vi "Status - Update Sequence Status.vi"(0 "Sequence Status":refnum<vi>, 1 "WPS Details":refnum<vi>, 2 "DB - Transaction":bool=TRUE, 3 "Transaction":T3, 5 "MCListBox FHS Setup":refnum<vi>, 7 "ET3504 Status":refnum<vi>, 11 "Error In":errorcluster, 12 "Parameter Cluster (Scaled)":T5={"ProgramNumber"=1, "CurProg"=33, "CurSeg"=1, "ProgStatus"=1, "ProgTimeLeft (min)"=0.0, "PVIn (degC)"=12000.0, "SPIn (NA)"=0.0, "SegTimeLeft (min)"=0.0}, 13 "DB - Active Process":bool=TRUE, 14 "Segment.Type":i16) -> (10 "Segment.Type II":i16, 15 "Error Out":errorcluster)   [LabVIEW 2013]
uses:
  Controls/Combo Box.ctl
  Controls/Transaction Cluster.ctl
  Controls/DB - Execute Transaction Enum.ctl
  Controls/DB - [TransactionResult] Enum.ctl
  Controls/DB - [Execute].[ActiveProcess] Enum.ctl
  Controls/DB - CMS Execute Active Process.ctl
  Controls/Global SRTRS.vi
panel:
  out "ET3504 Status":string="Offline."
  in  "WPS Details Setup 15":T2 caption="WPS Details"
  in  "MCListBox FHS Setup 2":i32(listbox) caption="Furnace Heating Sequence"
  out "Refnum error":errorcluster
  out "Seq-Seg Info":T4
  out "Sequence Status":string
  out "Total non-ZERO rows":i32
  # "Segment.Type\n0 - End\n1 - Rate\n3 - Dwell\n300 - mini Dwell"
  # "Segment.Type\n0 - End\n1 - Rate\n3 - Dwell"
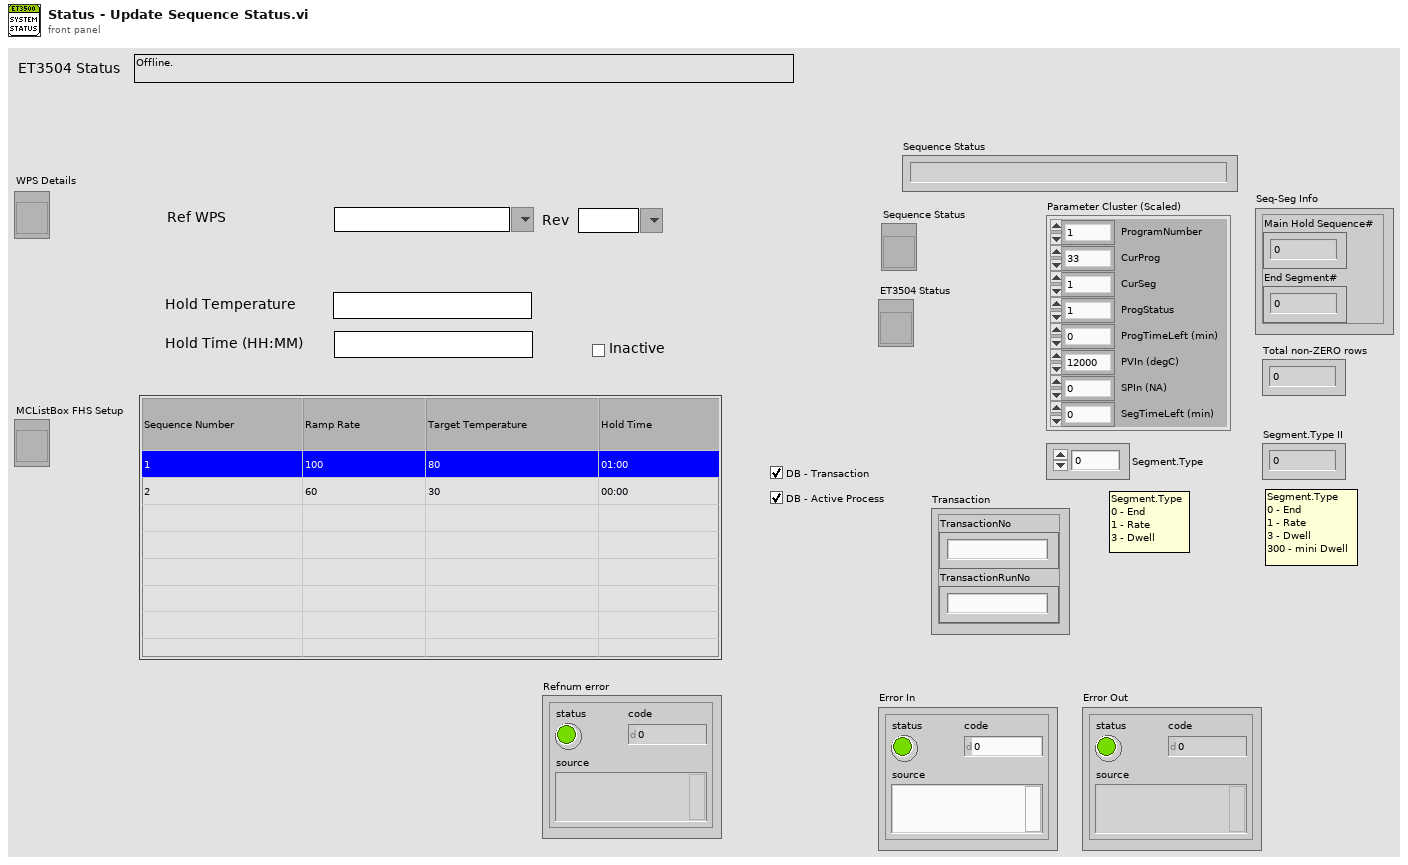
[diagram p1: front panel]
types:
  T1 = typedef "Combo Box.ctl" = string
  T2 = cluster{"WPS/Ref":T1, "Rev":T1, "Hold Temperature":string, "WPS Details Temperature Units":string, "Hold Time (HH:MM)":string, "Inactive":bool}
  T3 = typedef "Transaction Cluster.ctl" = cluster{"TransactionNo":string, "TransactionRunNo":string}
  T4 = cluster{"Main Hold Sequence#":i32, "End Segment#":i32}
  T5 = cluster{"ProgramNumber":i16, "CurProg":i16, "CurSeg":i16, "ProgStatus":i16, "ProgTimeLeft (min)":dbl, "PVIn (degC)":dbl, "SPIn (NA)":dbl, "SegTimeLeft (min)":dbl}
  T6 = typedef "Enum - InteractiveMode-SubVIMode.ctl" = enum16{"Interactive", "subVI Mode"}
  T7 = typedef "DB - Execute Transaction Enum.ctl" = enum16{"INSERT INTO [Header]", "INSERT INTO [TransactionResult]", "INSERT INTO [ProcedureItem]", "INSERT/UPDATE [Execute].[Active]", "SELECT [Execute].[Active]", "UPDATE [TransactionResult]", "UPDATE FILESTREAM", "SELECT [TransactionResult]", "SELECT [TransactionNo],[TransactionRunNo]"}
  T8 = typedef "DB - CMS Execute Active Process.ctl" = enum16{"INSERT INTO [Execute].[ActiveProcess]", "UPDATE [Execute].[ActiveProcess]", "SELECT [Execute].[ActiveProcess]", "UPDATE FILESTREAM", "SELECT FILESTREAM", "Check [IsActive]"}
  T9 = typedef "DB - [TransactionResult] Enum.ctl" = enum16{"[StartRecordTime]", "[StartRecordTemp]", "[MaxRecordedTemp]", "[MaxRecordedTempTime]", "[MinRecordedTemp]", "[MinRecordedTempTime]", "[EndRecordTemp]", "[EndRecordTime]", "[RecordedMinutes]", "[StartHoldTime]", "[StartHoldTemp]", "[HoldTimeMaxTemp]", "[HoldTimeMaxTempTime]", "[HoldTimeMinTemp]", "[HoldTimeMinTempTime]", "[EndHoldTime]", "[EndHoldTemp]", "[HoldDurationMinutes]", "[TempDiffDuringHold]", "[UnitOfTemperature]", "[PerformedBy]", "[PerformedOn]", "[IsTempWithinTol]", "[IsTimeWithinTol]", "[HoldTimePercentage]", "[ProcessStatus]", "[OverallStatus]", "[SequenceStatus]", "[Parameter1]", "[Parameter2]", "[Parameter3]", "[Parameter4]", "[Parameter5]", "[Parameter6]", "[Parameter7]", "[Parameter8]", "[Parameter9]", "[Parameter10]", "[Parameter11]", "[Parameter12]", "[Result]", "[RawDataFile]", "[RawDataFilePath]", "[RawDataFileName]", "[OutputSetId]", "[SavedBy]", "[SavedOn]", "[Inactive]"}
  T10 = typedef "DB - [Execute].[ActiveProcess] Enum.ctl" = enum16{"[IsActive]", "[TransactionNo]", "[TransactionRunNo]", "[SequenceStatus]", "[StartRecordTime]", "[EndRecordTime]", "[StartHoldTime]", "[EndHoldTime]", "[Message1]", "[Message2]", "[HoldTimeRemaining]", "[HoldTimePercentage]", "[HoldProgressColor]", "[OrderNumbers]", "[CurrentTemp]", "[UnitOfTemperature]", "[IsAppClientLive]", "[RawDataFile]", "[RecordedMinutes]", "[FurnaceControlStatus]", "[FurnaceControlColor]", "[ControllerStatus]", "[ControllerColor]", "[IsControllerOnline]", "[ProcessColor]", "[OverallColor]", "[LastUpdatedOn]", "[LastUpdatedCmsTime]", "[Inactive]"}
  T11 = typedef "DB - Logon Info.ctl" = cluster{"PlantID":string, "SystemID":string, "UserID":string, "DomainID":string, "LanguageID":string, "StationID":string}
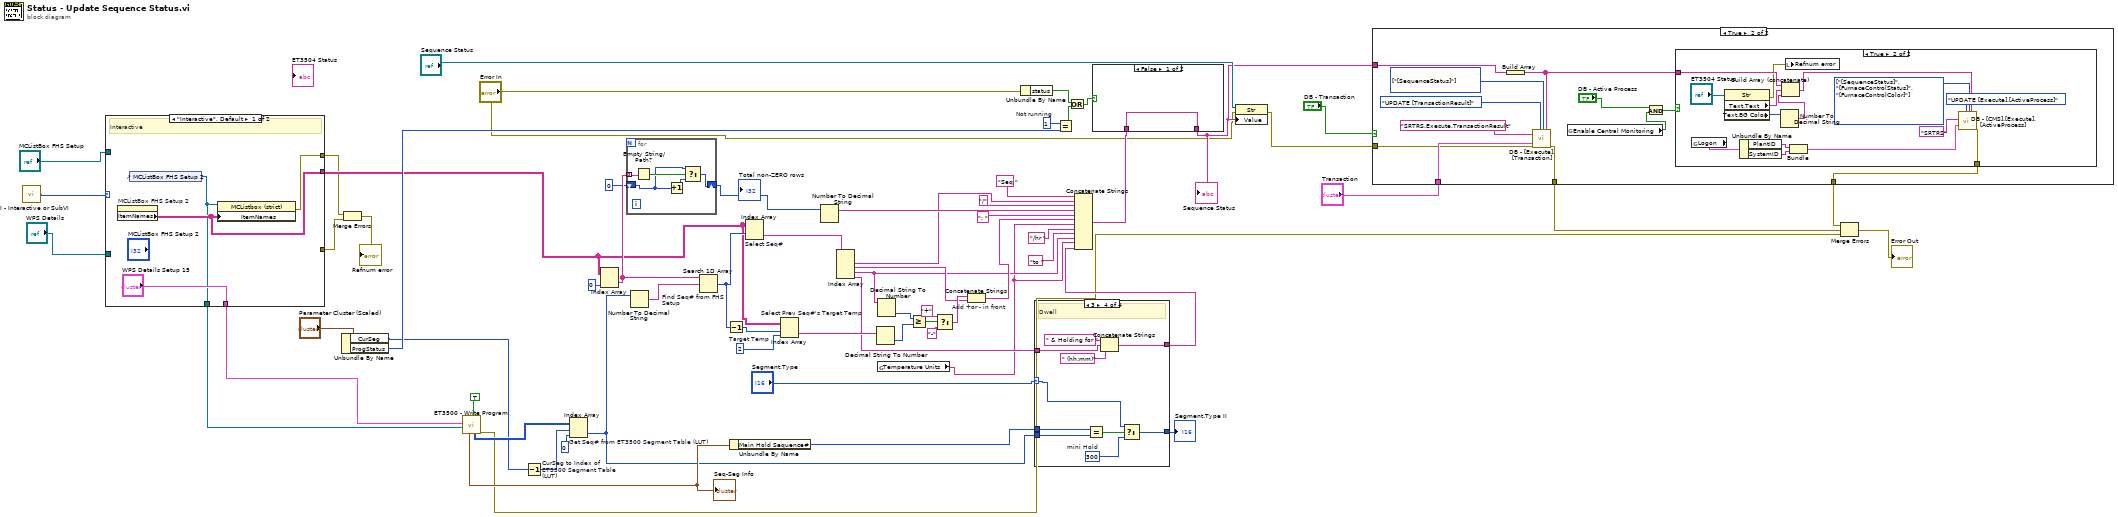
[diagram p0: block diagram]
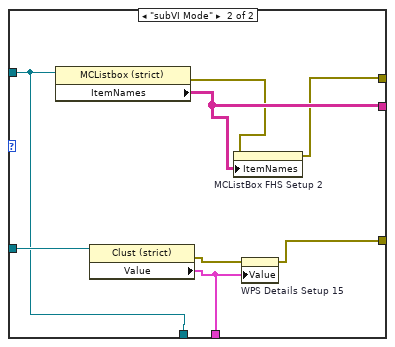
[diagram p2: hidden frame]
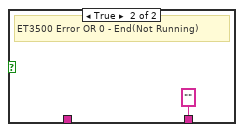
[diagram p5: hidden frame]
diagram:
  w37 = 2  # Target Temp
  w51 = i16 1  # Not running
  n1 = call "VI - Interactive or SubVI.vi"() -> ("Mode"=w2:T6)  [unwired: 5 in]
  n2 = case shown="\"Interactive\", Default" w2 {
    tunnel: "MCListBox FHS Setup" -> [_ w70]
    tunnel: [w69 w77] -> w11
    tunnel: [w68 w75] -> w7
    tunnel: "WPS Details" -> [_ w74]
    tunnel: ["WPS Details Setup 15" w72] -> w8
    tunnel: [_ w71] -> w5
    tunnel: [w66 w70] -> w1
    frame "Interactive", Default {
      # "Interactive"
      n3 = property on="MCListBox FHS Setup 2" class="MCListbox (strict)"() -> ("ItemNames"=w69:string[][])  [unwired: 2 in, 2 out]
      n4 = control-ref of="MCListBox FHS Setup 2"() -> (w66:refnum<vi>)
      n5 = property on="Property Node" class="MCListbox (strict)"(reference=w66, "ItemNames"=w69) -> (error out=w68:errorcluster)  [unwired: 1 in, 1 out]
    }
    frame "subVI Mode" {
      n6 = property on="Property Node" class="MCListbox (strict)"(reference=w70) -> (error out=w76:errorcluster, "ItemNames"=w77:string[][])  [unwired: 1 in, 1 out]
      n7 = property on="Property Node" class="Clust (strict)"(reference=w74) -> (error out=w73:errorcluster, "Value"=w72:T2)  [unwired: 1 in, 1 out]
      n8 = property on="MCListBox FHS Setup 2" class="MCListbox (strict)"(error in=w76, "ItemNames"=w77) -> (error out=w75:errorcluster)  [unwired: 1 in, 1 out]
      n9 = property on="WPS Details Setup 15" class="Clust (strict)"(error in=w73, "Value"=w72) -> (error out=w71:errorcluster)  [unwired: 1 in, 1 out]
    }
  }
  n10 = Unbundle By Name("Parameter Cluster (Scaled)") -> ("CurSeg"=w45:i16, "ProgStatus"=w50:i16)
  n11 = Merge Errors(w7, w5) -> (→"Refnum error":errorcluster)
  n12 = call "ET3500 - Write Program.vi"("Simulate"=TRUE, "MCListBox FHS Setup"=w1, "WPS Details Setup"=w8) -> ("ET3500"=w14:errorcluster, "ET3500 Segment Table"=w47:i32[][], "Seq-Seg Info"=w28:T4)  [unwired: 3 in, 3 out]
  "Seq-Seg Info" <- w28
  n13 = Decrement "CurSeg to Index of ET3500 Segment Table (LUT)"(x=w45) -> (x-1=w40:i16)
  n14 = Index Array "Get Seq# from ET3500 Segment Table (LUT)"(array=w47, index (row)=w40, index (col)=0 ("disabled index (col)")) -> (element=w26:i32)
  n15 = Index Array(array=w11, index (col)=0 ("disabled index (col)")) -> (element=w44:string[])  [unwired: 1 in]
  n16 = for {
    tunnel: w44 -> [w82] mode=indexing
    shift-right: [w78] -> w42
    shift-left: 0 -> [w79]
    n17 = Empty String/Path?(string/path=w82) -> (empty?=w81:bool)
    n18 = Increment(x=w79) -> (x+1=w80:i32)
    n19 = Select(t=w79, s=w81, f=w80) -> (s? t:f=w78:i32)
  }
  "Total non-ZERO rows" <- w42
  n20 = Number To Decimal String(number=w26) -> (decimal integer string=w59:string)  [unwired: 1 in]
  n21 = Search 1D Array "Find Seq# from FHS Setup"(1D array=w44, element=w59) -> (index of element=w39:i32)  [unwired: 1 in]
  n22 = Decrement(x=w39) -> (x-1=w38:i32)
  n23 = Unbundle By Name(w28) -> ("Main Hold Sequence#"=w27:i32)
  n24 = Index Array "Select Seq#"(array=w11, index (row)=w39) -> (element=w49:string[])  [unwired: 1 in]
  n25 = Index Array "Select Prev Seq#'s Target Temp"(array=w11, index (row)=w38, index (col)=w37) -> (element=w36:string)
  n26 = Number To Decimal String(number=w42) -> (decimal integer string=w62:string)  [unwired: 1 in]
  n27 = Index Array(array=w49) -> (element #1=w24:string, element #2=w23:string, element #3=w20:string, element #4=w30:string)  [unwired: 4 in]
  n28 = Decimal String To Number(string=w36) -> (number=w34:i32)  [unwired: 2 in, 1 out]
  n29 = Decimal String To Number(string=w20) -> (number=w35:i32)  [unwired: 2 in, 1 out]
  n30 = global read "Global SRTRS.vi" "Temperature Units"() -> (w4:string)
  n31 = Greater Or Equal?(x=w35, y=w34) -> (x >= y?=w33:bool)
  n32 = Select(t="+", s=w33, f="-") -> (s? t:f=w29:string)
  n33 = Concatenate Strings "Add +or - in front"(w29, w23) -> (w22:string)
  n34 = Unbundle By Name("Error In") -> ("status"=w54:bool)
  n35 = case shown="3" "Segment.Type" {
    selector: "Segment.Type" -> [w83 w84 w85 w88]
    tunnel: w30 -> [_ _ _ w94]
    tunnel: [_ _ _ w92] -> w41
    tunnel: w27 -> [_ _ _ w91]
    tunnel: w26 -> [_ _ _ w90]
    tunnel: [w83 w84 w85 w86] -> w25
    frame -1, Default {
      # "Undefined"
    }
    frame 0 {
      # "End"
    }
    frame 1 {
      # "Rate"
    }
    frame 3 {
      w87 = i16 300  # mini Hold
      # "Dwell"
      n36 = Equal?(x=w91, y=w90) -> (x = y?=w89:bool)
      n37 = Concatenate Strings(" & Holding for " ("string"), w94, " (hh:mm)" ("string")) -> (w92:string)
      n38 = Select(t=w88, s=w89, f=w87) -> (s? t:f=w86:i16)
    }
  }
  "Segment.Type II" <- w25
  n39 = Equal?(x=w51, y=w50) -> (x = y?=w53:bool)
  n40 = Or(x=w54, y=w53) -> (x .or. y?=w55:bool)
  n41 = Concatenate Strings("Seq " ("string"), w24, "/" ("string"), w62, ": " ("string"), w22, w4, "/hr " ("string"), "to " ("string"), w20, w4, w41) -> (w57:string)
  n42 = case shown="False" w55 {
    tunnel: w57 -> [w96 _]
    tunnel: [w96 ""] -> w17
    frame False {
    }
    frame True {
      # "ET3500 Error OR 0 - End(Not Running)"
    }
  }
  "Sequence Status" <- w17
  n43 = property on="Property Node" class="Str"(reference="Sequence Status", error in="Error In", "Value"=w17) -> (error out=w16:errorcluster)  [unwired: 1 out]
  n44 = case shown="True" "DB - Transaction" {
    tunnel: "Transaction" -> [_ w109]
    tunnel: w17 -> [_ w107]
    tunnel: w16 -> [w98 w105]
    tunnel: [w98 w104] -> w15
    tunnel: [_ w99] -> w3
    frame False {
    }
    frame True {
      w108 = T9[] [enum."[SequenceStatus]"] items=["[StartRecordTime]", "[StartRecordTemp]", "[MaxRecordedTemp]", "[MaxRecordedTempTime]", "[MinRecordedTemp]", "[MinRecordedTempTime]", "[EndRecordTemp]", "[EndRecordTime]", "[RecordedMinutes]", "[StartHoldTime]", "[StartHoldTemp]", "[HoldTimeMaxTemp]", "[HoldTimeMaxTempTime]", "[HoldTimeMinTemp]", "[HoldTimeMinTempTime]", "[EndHoldTime]", "[EndHoldTemp]", "[HoldDurationMinutes]", "[TempDiffDuringHold]", "[UnitOfTemperature]", "[PerformedBy]", "[PerformedOn]", "[IsTempWithinTol]", "[IsTimeWithinTol]", "[HoldTimePercentage]", "[ProcessStatus]", "[OverallStatus]", "[SequenceStatus]", "[Parameter1]", "[Parameter2]", "[Parameter3]", "[Parameter4]", "[Parameter5]", "[Parameter6]", "[Parameter7]", "[Parameter8]", "[Parameter9]", "[Parameter10]", "[Parameter11]", "[Parameter12]", "[Result]", "[RawDataFile]", "[RawDataFilePath]", "[RawDataFileName]", "[OutputSetId]", "[SavedBy]", "[SavedOn]", "[Inactive]"] ("[TransactionResult] v02")
      n45 = Build Array(w107) -> (w100:string[])
      n46 = call "DB - [Execute].[Transaction].vi"("DB.Schema.Table"="SRTRS.Execute.TransactionResult", "Transaction"=w109, "error in (no error)"=w105, "DB - Execute Transaction"=DB_-_Execute_Transaction_Enum."UPDATE [TransactionResult]" ("DB - Setup Item Enum"), "[TransactionResult] v02"=w108, "<Values>"=w100) -> ("SUMMARY"=w104:errorcluster)  [unwired: 10 in, 3 out]
      n47 = global read "Global SRTRS.vi" "Enable Central Monitoring"() -> (w101:bool)
      n48 = And(x="DB - Active Process", y=w101) -> (x .and. y?=w102:bool)
      n49 = case shown="True" w102 {
        tunnel: w100 -> [_ w116]
        tunnel: [_ w121] -> w99
        frame False {
        }
        frame True {
          w125 = T10[] [enum."[SequenceStatus]", enum."[FurnaceControlStatus]", enum."[FurnaceControlColor]"] items=["[IsActive]", "[TransactionNo]", "[TransactionRunNo]", "[SequenceStatus]", "[StartRecordTime]", "[EndRecordTime]", "[StartHoldTime]", "[EndHoldTime]", "[Message1]", "[Message2]", "[HoldTimeRemaining]", "[HoldTimePercentage]", "[HoldProgressColor]", "[OrderNumbers]", "[CurrentTemp]", "[UnitOfTemperature]", "[IsAppClientLive]", "[RawDataFile]", "[RecordedMinutes]", "[FurnaceControlStatus]", "[FurnaceControlColor]", "[ControllerStatus]", "[ControllerColor]", "[IsControllerOnline]", "[ProcessColor]", "[OverallColor]", "[LastUpdatedOn]", "[LastUpdatedCmsTime]", "[Inactive]"] ("[Execute].[ActiveProcess]\n2014-10-14 14:58")
          n50 = global read "Global SRTRS.vi" "Logon"() -> (w124:T11)
          n51 = property class="Str"(reference="ET3504 Status") -> (error out=w113:errorcluster, "Text.Text"=w119:string, "Text.BG Color"=w118:u32)  [unwired: 1 in, 1 out]
          n52 = Unbundle By Name(w124) -> ("PlantID"=w123:string, "SystemID"=w122:string)
          n53 = Number To Decimal String(number=w118) -> (decimal integer string=w117:string)  [unwired: 1 in]
          n54 = Build Array (concatenate)(w116, w119, w117) -> (w115:string[])
          n55 = local write "Refnum error"(w113) -> ()
          n56 = Bundle("PlantID"=w123, "SystemID"=w122) -> (w114:cluster{"PlantID":string, "SystemID":string})  [unwired: 1 in]
          n57 = call "DB - [CMS].[Execute].[ActiveProcess].vi"("Application"="SRTRS", "[PlantId],[SystemId]"=w114, "DB - CMS Execute ActiveProcess"=DB_-_CMS_Execute_Active_Process."UPDATE [Execute].[ActiveProcess]", "[Execute].[ActiveProcess]\n2014-10-14 14:58"=w125, "<Data>"=w115) -> ("SUMMARY"=w121:errorcluster)  [unwired: 11 in, 3 out]
        }
      }
    }
  }
  n58 = Merge Errors(w3, w15, w14) -> (→"Error Out":errorcluster)
